vi "CLSUIP_FindClassControlOrIndicator.vi"(3 "error in (no error)":errorcluster, 4 "Indicator?":bool, 5 "VI Refnum":refnum<vi>) -> (0 "error out":errorcluster, 1 "LVClassControl Refnum":refnum<vi>, 2 "VI Refnum out":refnum<vi>)   [LabVIEW 2021, in "MemberVICreation.lvlib"]
uses:
  <resource>/Framework/Providers/LVClassLibrary/NewAccessors/MemberVICreation.lvlib
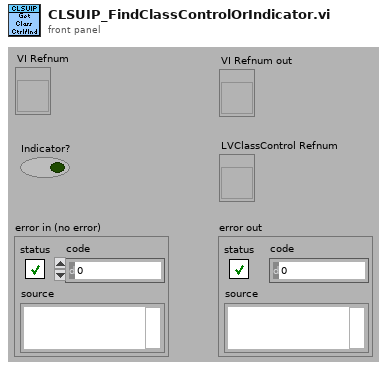
[diagram p1: front panel]
types:
  T1 = typedef "LVRectTypeDef.ctl" = cluster{"left":i16, "top":i16, "right":i16, "bottom":i16}
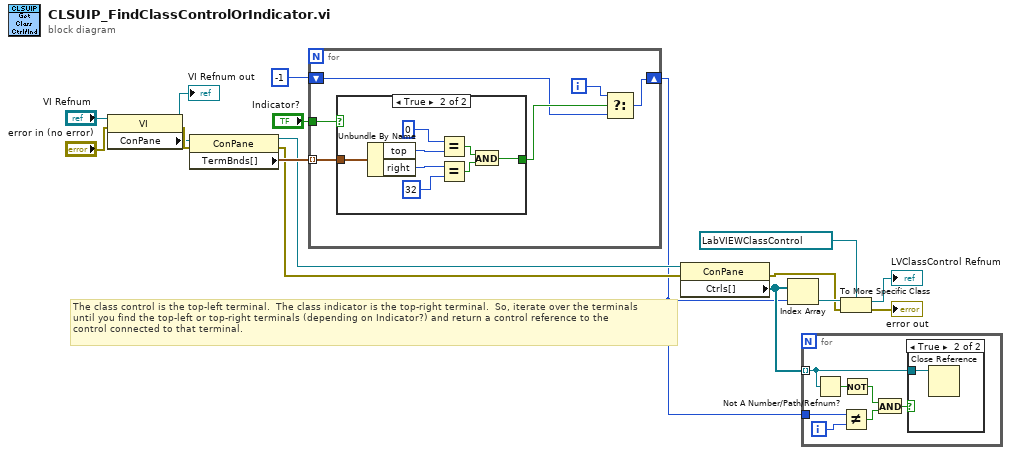
[diagram p0: block diagram]
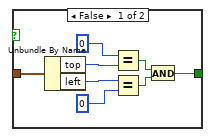
[diagram p3: hidden frame]
diagram:
  # "The class control is the top-left terminal.  The class indicator is the top-right terminal.  So, iterate over the terminals\nuntil you find the top-left or top-right terminals (depending on Indicator?) and return a control reference to the\ncontrol connected to that terminal."
  n1 = property class="VI"(reference="VI Refnum", error in="error in (no error)") -> (reference out=→"VI Refnum out":refnum<vi>, error out=w16:errorcluster, "ConPane"=w15:refnum<vi>)
  n2 = property class="ConPane"(reference=w15, error in=w16) -> (reference out=w9:refnum<vi>, error out=w10:errorcluster, "TermBnds[]"=w14:T1[])
  n3 = for {
    tunnel: w14 -> [w22] mode=indexing
    shift-right: [w18] -> w7
    shift-left: -1 -> [w19]
    tunnel: "Indicator?" -> [w23]
    i -> [w20]
    n4 = case shown="True" w23 {
      tunnel: w22 -> [w27 w39]
      tunnel: [w24 w32] -> w21
      frame False {
        n5 = Unbundle By Name(w27) -> ("top"=w31:i16, "left"=w30:i16)
        n6 = Equal?(x=i16 0, y=w31) -> (x = y?=w25:bool)
        n7 = Equal?(x=w30, y=i16 0) -> (x = y?=w26:bool)
        n8 = And(x=w25, y=w26) -> (x .and. y?=w24:bool)
      }
      frame True {
        n9 = Unbundle By Name(w39) -> ("top"=w38:i16, "right"=w37:i16)
        n10 = Equal?(x=i16 0, y=w38) -> (x = y?=w34:bool)
        n11 = Equal?(x=w37, y=i16 32) -> (x = y?=w33:bool)
        n12 = And(x=w34, y=w33) -> (x .and. y?=w32:bool)
      }
    }
    n13 = Select(t=w20, s=w21, f=w19) -> (s? t:f=w18:i32)
  }
  n14 = property class="ConPane"(reference=w9, error in=w10) -> (error out=w2:errorcluster, "Ctrls[]"=w8:refnum<vi>[])  [unwired: 1 out]
  n15 = Index Array(array=w8, index=w7) -> (element=w6:refnum<vi>)
  n16 = for {
    tunnel: w8 -> [w43] mode=indexing
    tunnel: w7 -> [w44]
    i -> [w46]
    n17 = Not A Number/Path/Refnum?(number/path/refnum=w43) -> (NaN/Path/Refnum?=w41:bool)
    n18 = Not Equal?(x=w44, y=w46) -> (x != y?=w45:bool)
    n19 = Not(x=w41) -> (.not. x?=w40:bool)
    n20 = And(x=w40, y=w45) -> (x .and. y?=w42:bool)
    n21 = case shown="True" w42 {
      tunnel: w43 -> [_ w47]
      frame False {
      }
      frame True {
        n22 = Close Reference(reference=w47) -> ()  [unwired: 1 in, 1 out]
      }
    }
  }
  n23 = To More Specific Class(target class=refnum<vi> refnum ("LVClassControl Refnum 2"), reference=w6, error in=w2) -> (specific class reference=→"LVClassControl Refnum":refnum<vi>, error out=→"error out":errorcluster)
